vi "Host_Laser.vi"() -> ()   [LabVIEW 2018]
uses:
  <vilib>/userdefined/High Color/nirio_resource_hc.ctl
  C:/LabView_PRJ/EV76C661/Spels.AutomationTools.RemoteFunctionalControlService.dll
  Spels.AutomationTools.RemoteFunctionalControlService.dll
  <instrlib>/niDCPower/nidcpower.llb/niDCPower Measurement Type.ctl
  <vilib>/FPGAPlugInAG/PXI-7953R/niLvFpga_Open_PXI-7953R.vi
  <vilib>/rvi/interface/common/dynamic/niFpgaDynamicAddResources.vi
  <vilib>/FPGAPlugInAG/Dynamic/niLvFpga_Reset_Dynamic.vi
  <vilib>/FPGAPlugInAG/Dynamic/niLvFpga_Run_Dynamic.vi
  <vilib>/Utility/error.llb/Error Cluster From Error Code.vi
  <vilib>/rvi/errors/niLvFpgaAdjustHostInterfaceError.vi
  <vilib>/FPGAPlugInAG/Dynamic/niLvFpga_Abort_Dynamic.vi
  <vilib>/rvi/interface/nirviOpenFPGA/nirviOpenFPGA.xnode
  FPGA Bitfiles/EV76C661_FPGATarget_Target_LxE3WAGXilk.lvbitx
  <vilib>/rvi/interface/nirviMethod/nirviMethod.xnode
  <vilib>/rvi/interface/nirviReadWriteControl/nirviReadWriteControl.xnode
  NiFpgaLv.dll
  <vilib>/rvi/interface/Simulation/niFpgaSimulationCallBeginRW.vi
  <vilib>/FPGAPlugInAG/Dynamic/niLvFpga_ReadFifo_Dynamic.vi
  <vilib>/rvi/errors/niLvFpgaMergeErrorWithErrorCode.vi
panel:
  out "Data":string
  out "Image":T1(plugin-control)
  in  "Содержание всех регистров":u32[](array[numeric])=[1, 0, 0, 0, 32880, 0, 53338, 2561, 56217, 24976, 512, 260, 0, 0, 512, 0, 0, 0, 6, 1024, 6, 1280, 0, 0, 0, 0, 0, 512, 0, 0, 0, 6, 1024, 6, 1280, 0, 512, 0, 0, 0, 6, 1024, 6, 1280, 0, 512, 0, 0, 0, 6, 1024, 6, 1280, 0, 32896, 32896, 0, 14464, 32960, 0, 0, 0, 0, 0, 0, 0, 0, 0, 8192, 0, 0, 0, 0, 31601, 0, 0, 0, 0, 0, 0, 0, 0, 0, 0, 0, 0, 0, 0, 0, 0, 0, 0, 0, 0, 0, 0, 0, 0, 0, 0, 0, 0, 0, 0, 0, 0, 0, 0, 0, 0, 0, 0, 0, 0, 0, 0, 0, 0, 0, 0, 0, 0, 0, 0, 0, 0, 0, 2048]
  in  "Запись 6 регистров":u32[](array[numeric])=[2561, 56217, 24976, 512, 260, 512]
  in  "SPI_прошить":bool
  out "ST":bool
  in  "RESET":bool
  in  "Автомат":bool
  in  "VDD33_ON":bool
  in  "VDD18_ON":bool
  in  "Светлый (T)\nТемный (F)":bool
  in  "Frames":path=path "C:/LabView_PRJ/EV76C661/FRAMES"
  in  "ПРИМЕЧАНИЕ":string
  in  "SAVE":bool
  in  "Получить кадр":bool
  out "Data":u8[][](array[numeric])
  in  "Непрерывно":bool
  out "Сбои":i32
  out "СБОЙ":string="ОК"
  out "СБОЙ!":bool
  out "ПОСЛЕДНИЙ СБОЙ":string="0"
  out "COUNT":u8
  out "SPI_OUT":bool[](array[boolean])
  in  "МАСКИРУЕМ":i32[](array[numeric])=[0, -1, 2, 3, 4, 5, 6, 7, 8, 9, 10, 11, 12, 13, 14, 15, 16, 17, 18, 19, 20, 21, 22, 23, 24, 25, 26, 27, 28, 29, 30, 31, 32, 33, 34, 35, 36, 37, 38, 39, 40, 41, 42, 43, 44, 45, 46, 47, 48, 49, 50, 51, 52, 53, 54, 55, 56, 57, 58, 59, -1, -1, -1, -1, -1, -1, -1, -1, -1, -1, -1, -1, -1, -1, -1, -1, -1, -1, -1, -1, -1, -1, -1, -1, -1, -1, -1, -1, -1, -1, -1, -1, -1, -1, -1, -1, -1, -1, -1, -1, -1, -1, -1, -1, -1, -1, -1, -1, -1, -1, -1, -1, -1, -1, -1, -1, -1, -1, -1, -1, -1, -1, -1, -1, -1, -1, -1, 127, 0, 0, 0, 0, 0, 0, 0, 0, 0, 0, 0, 0, 0, 0, 0, 0, 0, 0, 0, 0, 0, 0, 0, 0, 0, 0, 0, 0, 0, 0, 0, 0, 0, 0, 0, 0, 0, 0, 0, 0, 0, 0, 0, 0, 0, 0, 0, 0, 0, 0, 0, 0, 0, 0, 0, 0, 0, 0, 0, 0, 0, 0, 0, 0, 0, 0, 0, 0, 0, 0, 0, 0, 0, 0, 0, 0, 0, 0, 0, 0, 0, 0, 0, 0, 0, 0, 0, 0, 0, 0, 0, 0, 0, 0, 0, 0, 0, 0, 0, 0, 0, 0, 0, 0, 0, 0, 0, 0, 0, 0, 0, 0, 0, 0, 0, 0, 0, 0, 0, 0, 0, 0, 0, 0, 0, 0, 0, 0]
  in  "ПРОВЕРКА СБОЕВ?":bool
  out "GC":u8
  out "REG_WR":bool
  in  "SIM_SEL":bool
  out "SEL":bool
  in  "VDD18A_selcur":dbl=0.05 caption="current limit" format="%_6p"
  in  "VDD33A_selcur":dbl=0.035 caption="current limit" format="%_6p"
  in  "VDD18D_selcur":dbl=0.055 caption="current limit" format="%_6p"
  out "VDD18A":i32
  out "VDD18A":bool
  out "VDD33A":i32
  out "VDD33A":bool
  out "VDD18D":i32
  out "VDD18D":bool
  in  "VDD18A, V":dbl=1.8 caption="voltage level" format="%_6p"
  in  "VDD18A_curlim, A":dbl=0.1 caption="current limit" format="%_6p"
  in  "VDD33A_curlim, A":dbl=0.1 caption="current limit" format="%_6p"
  out "VDD18A_cur, A":dbl caption="measurement" format="%_6g"
  out "VDD33A_cur, A":dbl caption="measurement" format="%_6g"
  in  "VDD33A, V":dbl=3.3 caption="voltage level" format="%_6p"
  in  "VDD18D, V":dbl=1.8 caption="voltage level" format="%_6p"
  in  "VDD18D_curlim, A":dbl=0.1 caption="current limit" format="%_6p"
  out "VDD18D_cur, A":dbl caption="measurement" format="%_6g"
  in  "Питание":bool
  out "VDD33A Chart":dbl(graph)=0.0006520018718277456
  out "VDD18D Chart":dbl(graph)=-6.889343232631937
  out "VDD18A Chart":dbl(graph)=0.09491557293549348 caption="Waveform Chart 5"
  in  "Стоп":bool
  in  "VDD18A_33A":refnum<k15>="PXI1Slot2" caption="instrument handle"
  in  "VDD18D":refnum<k15>="PXI1Slot3" caption="instrument handle"
  in  "resource name":T2="PXI1Slot6"
  in  "SEU":path=path "C:/LabView_PRJ/EV76C661/SEU"
  in  "SEL":path=path "C:/LabView_PRJ/EV76C661/SEL"
  out "Номер образца":string="0"
  # "1,6/1,8/2,0"
  # "3,15/3,3/3,45"
  # "h07, h08, h09, h0A, h0B, h0E"
  # "h0E - отвечает за экспозицию\nОт 1 до 65535"
  # "1,6/1,8/2,0"
  # "0"
  # "1"
  # "2"
  # "3"
  # "4"
  # "5"
  # "6"
  # "7"
  # "8"
  # "9"
  # "10"
  # "11"
  # "12"
  # "13"
  # "14"
  # "15"
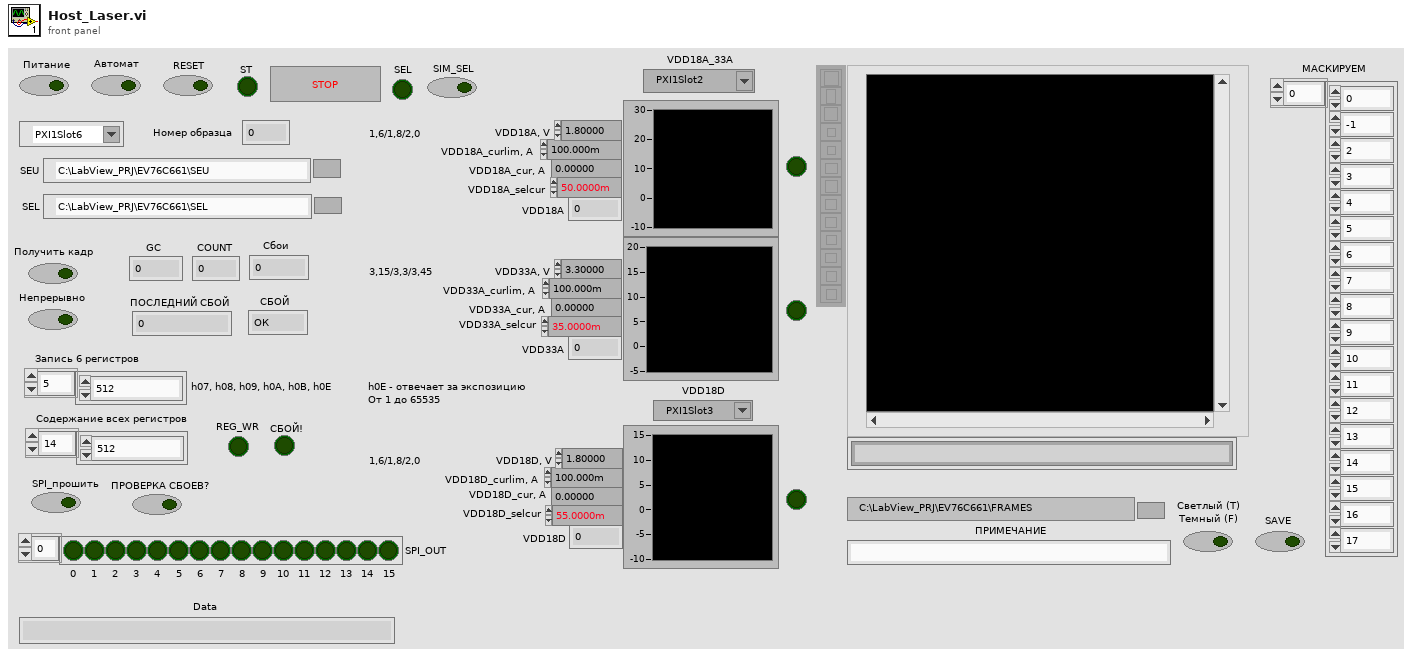
[diagram p1: front panel]
types:
  T1 = typedef "IMAQ Image.ctl" = refnum<image>
  T2 = typedef "nirio_resource_hc.ctl" = tag
  T3 = typedef "Image Type" = u32
  T4 = enum16{"open", "replace", "create", "open or create", "replace or create", "replace or create with confirmation"}
  T5 = typedef "niDCPower Measurement Type.ctl" = i32
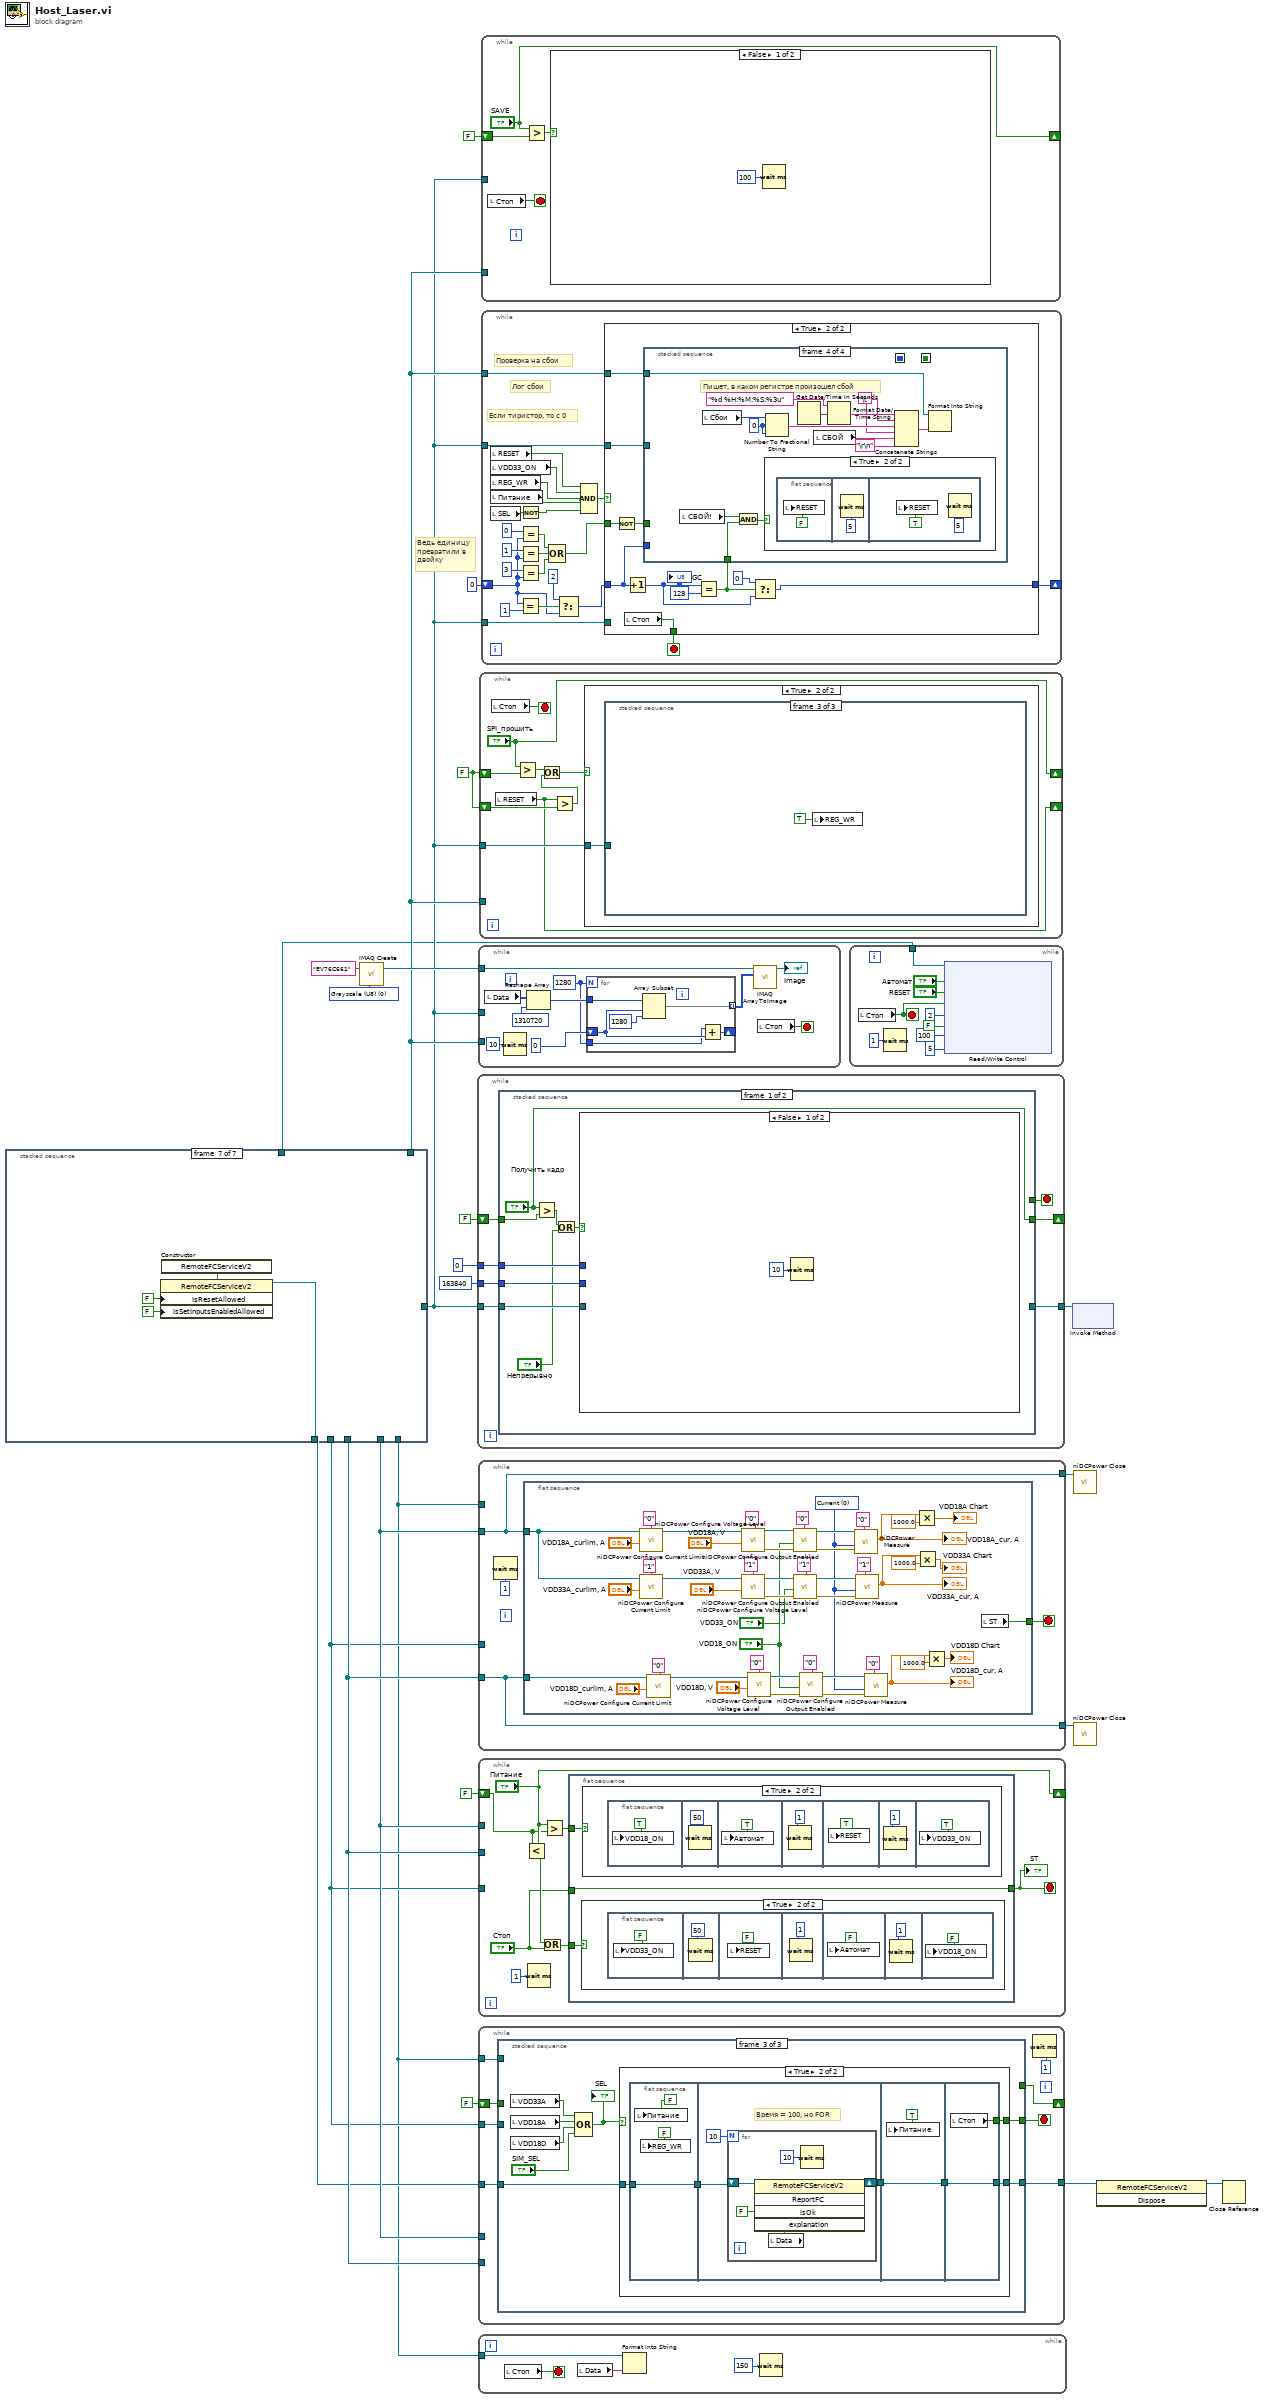
[diagram p0: block diagram]
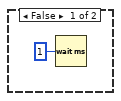
[diagram p2: hidden frame]
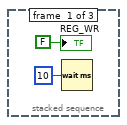
[diagram p3: hidden frame]
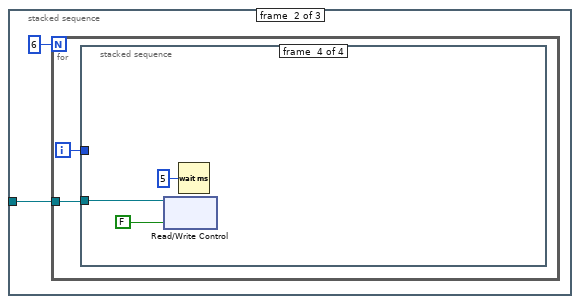
[diagram p4: hidden frame]
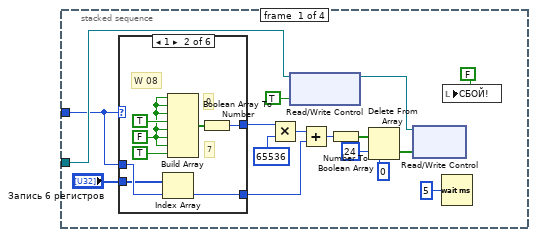
[diagram p5: hidden frame]
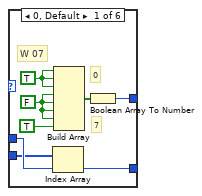
[diagram p6: hidden frame]
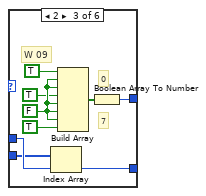
[diagram p7: hidden frame]
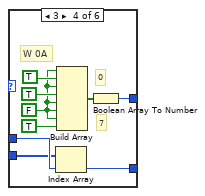
[diagram p8: hidden frame]
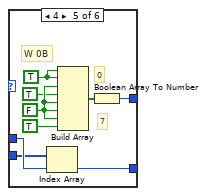
[diagram p9: hidden frame]
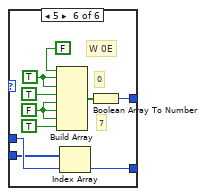
[diagram p10: hidden frame]
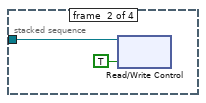
[diagram p11: hidden frame]
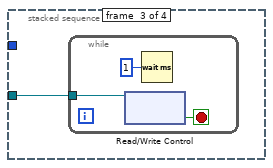
[diagram p12: hidden frame]
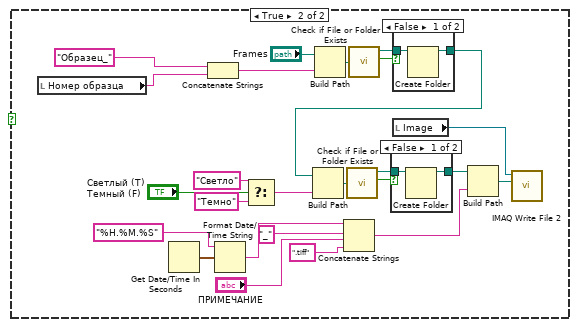
[diagram p15: hidden frame]
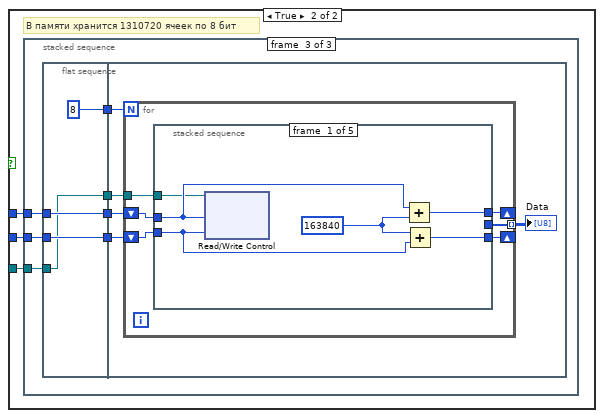
[diagram p18: hidden frame]
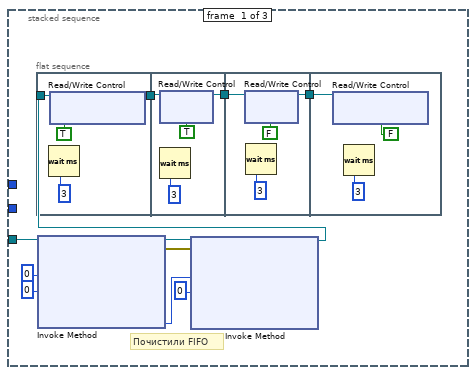
[diagram p19: hidden frame]
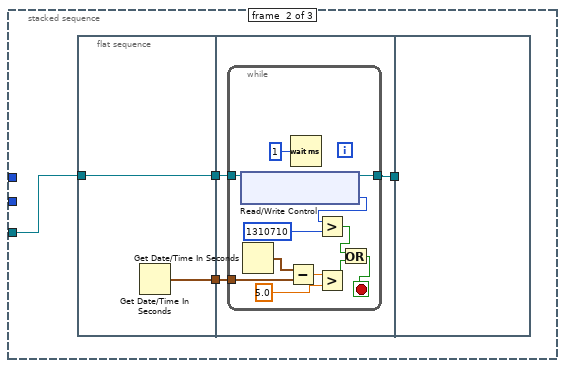
[diagram p20: hidden frame]
diagram:
  w7 = FALSE
  w19 = T3 0 items=["Grayscale (U8)", "Grayscale (I16)", "Grayscale (SGL)", "Complex (CSG)", "RGB (U32)", "HSL (U32)", "RGB (U64)"] ("Image Type")
  # "Ведь единицу \nпревратили в \nдвойку"
  n1 = stacked-sequence {
    tunnel: [_ _ _ _ w95 _ _] -> w6
    tunnel: [_ _ _ _ _ w102 _] -> w12
    tunnel: [_ _ _ _ _ w101 _] -> w11
    tunnel: [_ _ w40 _ _ _ _] -> w3
    tunnel: [_ _ _ _ w95 _ _] -> w10
    tunnel: [_ _ _ w66 _ _ _] -> w9
    tunnel: [_ _ _ _ w95 _ _] -> w5
    tunnel: [_ _ _ _ _ _ w113] -> w4
    frame #0 {
      n2 = call "Begin.vi"() -> ("Номер образца 2"=→"Номер образца":string)  [unwired: 11 in]
    }
    frame #1 {
      w29 = 0
      w30 = ""
      w26 = FALSE
      n3 = local write "ПОСЛЕДНИЙ СБОЙ"(w30) -> ()
      n4 = local write "СБОЙ"(w30) -> ()
      n5 = local write "Сбои"(w29) -> ()
      n6 = local write "VDD18A"(w29) -> ()
      n7 = local write "VDD33A"(w29) -> ()
      n8 = local write "VDD18D"(w29) -> ()
      n9 = local write "GC"(u8 0 ("GC")) -> ()
      n10 = local write "COUNT"(u16 0 ("COUNT")) -> ()
      n11 = local write "RESET"(w26) -> ()
      n12 = local write "SPI_прошить"(w26) -> ()
      n13 = local write "REG_WR"(w26) -> ()
      n14 = local write "Непрерывно"(w26) -> ()
      n15 = local write "Получить кадр"(w26) -> ()
      n16 = local write "VDD18A"(w26) -> ()
      n17 = local write "VDD33A"(w26) -> ()
      n18 = local write "VDD18D"(w26) -> ()
      n19 = local write "ST"(w26) -> ()
      n20 = local write "SEL"(w26) -> ()
      n21 = local write "Питание"(w26) -> ()
      n22 = local write "Стоп"(w26) -> ()
      n23 = local write "СБОЙ!"(w26) -> ()
      n24 = local write "SAVE"(w26) -> ()
      n25 = local write "ПРОВЕРКА СБОЕВ?"(w26) -> ()
      n26 = local write "Автомат"(w26) -> ()
      n27 = local write "SIM_SEL"(w26) -> ()
      n28 = local write "VDD18_ON"(w26) -> ()
      n29 = local write "VDD33_ON"(w26) -> ()
    }
    frame #2 {
      w41 = "\t"
      # "Инициализаци первой строки лога по токам"
      n30 = local read "Номер образца"() -> (w53:string)
      n31 = Build Path(base path="SEL", name or relative path=w53) -> (appended path=w55:path)
      n32 = Get Date/Time In Seconds() -> (seconds since 1Jan1904=w48:timestamp)
      n33 = call <vilib>:"Check if File or Folder Exists.vi"("path"=w55) -> ("file or folder exists?"=w56:bool, "dup path"=w57:path)  [unwired: 8 in, 1 out]
      n34 = Format Date/Time String(time format string (%c)="%d %H.%M.%S", seconds (now)=w48) -> (date/time string=w45:string)  [unwired: 1 in]
      n35 = case shown="False" w56 {
        tunnel: w57 -> [w63 w64]
        tunnel: [w62 w64] -> w39
        frame False {
          n36 = Create Folder(path (use dialog)=w63) -> (created path=w62:path)  [unwired: 2 in, 2 out]
        }
        frame True {
        }
      }
      n37 = Concatenate Strings(w45, ".xls" ("string")) -> (w43:string)
      n38 = Build Path(base path=w39, name or relative path=w43) -> (appended path=w46:path)
      n39 = Open/Create/Replace File(file path (use dialog)=w46, operation (0:open)=T4."open or create", access (0:read/write)=enum16{"read/write", "read-only", "write-only"}."read/write") -> (refnum out=w49:refnum<file>)  [unwired: 3 in, 2 out]
      n40 = case shown="True" TRUE {
        tunnel: w49 -> [w58 w61]
        tunnel: [w58 w59] -> w42
        frame False {
        }
        frame True {
          n41 = Set File Position(refnum=w61, from (0:start)=enum16{"start", "end", "current"}."end") -> (refnum out=w59:refnum<file>)  [unwired: 2 in, 1 out]
        }
      }
      n42 = Format Into String(initial string=w42, "Time" ("input 1"), w41, "V_18A_cur" ("input 1"), w41, "V_33A_cur" ("input 1"), w41, "V_18D_cur" ("input 1"), w41, "V_18A_sel" ("input 1"), w41, "V_33A_sel" ("input 1"), w41, "V_18D_sel" ("input 1"), "\r\n") -> (resulting string=w40:refnum<file>)  [unwired: 2 in, 1 out]
    }
    frame #3 {
      w75 = "\t"
      n43 = local read "Номер образца"() -> (w83:string)
      n44 = Build Path(base path="SEU", name or relative path=w83) -> (appended path=w85:path)
      n45 = Get Date/Time In Seconds() -> (seconds since 1Jan1904=w81:timestamp)
      n46 = call <vilib>:"Check if File or Folder Exists.vi"("path"=w85) -> ("file or folder exists?"=w86:bool, "dup path"=w87:path)  [unwired: 8 in, 1 out]
      n47 = Format Date/Time String(time format string (%c)="%d %H.%M.%S", seconds (now)=w81) -> (date/time string=w79:string)  [unwired: 1 in]
      n48 = case shown="False" w86 {
        tunnel: w87 -> [w93 w94]
        tunnel: [w92 w94] -> w65
        frame False {
          n49 = Create Folder(path (use dialog)=w93) -> (created path=w92:path)  [unwired: 2 in, 2 out]
        }
        frame True {
        }
      }
      n50 = Concatenate Strings(w79, ".xls" ("string")) -> (w78:string)
      n51 = Build Path(base path=w65, name or relative path=w78) -> (appended path=w80:path)
      n52 = Open/Create/Replace File(file path (use dialog)=w80, operation (0:open)=T4."open or create", access (0:read/write)=enum16{"read/write", "read-only", "write-only"}."read/write") -> (refnum out=w82:refnum<file>)  [unwired: 3 in, 2 out]
      n53 = case shown="True" TRUE {
        tunnel: w82 -> [w88 w91]
        tunnel: [w88 w89] -> w77
        frame False {
        }
        frame True {
          n54 = Set File Position(refnum=w91, from (0:start)=enum16{"start", "end", "current"}."end") -> (refnum out=w89:refnum<file>)  [unwired: 2 in, 1 out]
        }
      }
      n55 = Format Into String(initial string=w77, "Time" ("input 1"), w75, "Count" ("input 3"), w75, "#reg" ("input 5"), "\r\n") -> (resulting string=w66:refnum<file>)  [unwired: 2 in, 1 out]
    }
    frame #4 {
      n56 = xnode "Open FPGA VI Reference"("resource name"="resource name") -> ("FPGA VI Reference Out"=w100:refnum<k20>, "error out"=w98:errorcluster)  [unwired: 1 in]
      n57 = xnode "Invoke Method"("FPGA VI Reference In"=w100, "error in"=w98) -> ("FPGA VI Reference Out"=w97:refnum<k20>, "error out"=w99:errorcluster)
      n58 = xnode "Invoke Method"("FPGA VI Reference In"=w97, "error in"=w99) -> ("FPGA VI Reference Out"=w95:refnum<k20>)  [unwired: 1 in, 1 out]
    }
    frame #5 {
      n59 = call <instrlib>:"niDCPower Initialize.vi"("resource name"="VDD18A_33A") -> ("error out"=w109:errorcluster, "instrument handle out"=w111:refnum<k15>)  [unwired: 3 in, 6 out]
      n60 = call <instrlib>:"niDCPower Initialize.vi"("resource name"="VDD18D") -> ("error out"=w110:errorcluster, "instrument handle out"=w112:refnum<k15>)  [unwired: 3 in, 6 out]
      n61 = call <instrlib>:"niDCPower Configure Voltage Level.vi"("error in (no error)"=w109, "voltage level"=0.0, "channel name"="0,1", "instrument handle"=w111) -> ("instrument handle out"=w101:refnum<k15>)  [unwired: 6 in, 1 out]
      n62 = call <instrlib>:"niDCPower Configure Voltage Level.vi"("error in (no error)"=w110, "voltage level"=0.0, "channel name"="0", "instrument handle"=w112) -> ("instrument handle out"=w102:refnum<k15>)  [unwired: 6 in, 1 out]
    }
    frame #6 {
      n63 = constructor class="RemoteFCServiceV2"() -> (reference out=w116:refnum<k24>)  [unwired: 3 in, 2 out]
      n64 = property class="RemoteFCServiceV2"(reference=w116, "IsResetAllowed"=FALSE, "IsSetInputsEnabledAllowed"=FALSE) -> (reference out=w113:refnum<k24>)  [unwired: 1 in, 1 out]
    }
  }
  n65 = call "IMAQ Create"("Image Name"="EV76C661", "Image Type"=w19) -> ("New Image"=w18:T1)  [unwired: 3 in, 1 out]
  n66 = while {
    tunnel: w6 -> [w123]
    tunnel: [w122] -> w24
    tunnel: u32 163840 ("163840") -> [w121]
    tunnel: u32 0 -> [w119]
    shift-right: [w117] -> _
    shift-left: FALSE ("Получить кадр") -> [w118]
    stop <- w120 stop-if-true
    n67 = stacked-sequence {
      tunnel: w123 -> [w130 w227]
      tunnel: [_ w227] -> w122
      tunnel: w121 -> [w131 _]
      tunnel: [_ w226] -> w120
      tunnel: w119 -> [w129 _]
      tunnel: w118 -> [w128 _]
      tunnel: ["Получить кадр" _] -> w117
      frame #0 {
        n68 = Greater?(x="Получить кадр", y=w128) -> (0:w127:bool)
        n69 = Or(x=w127, y="Непрерывно") -> (x .or. y?=w125:bool)
        n70 = case shown="False" w125 {
          tunnel: w130 -> [_ w135]
          tunnel: w131 -> [_ w134]
          tunnel: w129 -> [_ w133]
          frame False {
            n71 = Wait (ms)(milliseconds to wait=u32 10) -> ()  [unwired: 1 out]
          }
          frame True {
            # "В памяти хранится 1310720 ячеек по 8 бит"
            n72 = stacked-sequence {
              tunnel: w135 -> [w140 w163 w189]
              tunnel: w134 -> [_ _ w185]
              tunnel: w133 -> [_ _ w187]
              frame #0 {
                # "Почистили FIFO"
                n73 = flat-sequence {
                  tunnel: w138 -> [w150]
                  tunnel: [w147] -> w139
                  tunnel: w139 -> [w152]
                  tunnel: [w151] -> w137
                  tunnel: w137 -> [w158]
                  tunnel: [w157] -> w136
                  tunnel: w136 -> [w161]
                  frame #0 {
                    n74 = Wait (ms)(milliseconds to wait=u32 3) -> ()  [unwired: 1 out]
                    n75 = xnode "Read/Write Control"("FPGA VI Reference In"=w150, "Кадр в память"=TRUE) -> ("FPGA VI Reference Out"=w147:refnum<k20>)  [unwired: 1 in, 1 out]
                  }
                  frame #1 {
                    n76 = xnode "Read/Write Control"("FPGA VI Reference In"=w152, "TRIG"=TRUE ("Кадр в память")) -> ("FPGA VI Reference Out"=w151:refnum<k20>)  [unwired: 1 in, 1 out]
                    n77 = Wait (ms)(milliseconds to wait=u32 3) -> ()  [unwired: 1 out]
                  }
                  frame #2 {
                    n78 = xnode "Read/Write Control"("FPGA VI Reference In"=w158, "TRIG"=FALSE) -> ("FPGA VI Reference Out"=w157:refnum<k20>)  [unwired: 1 in, 1 out]
                    n79 = Wait (ms)(milliseconds to wait=u32 3) -> ()  [unwired: 1 out]
                  }
                  frame #3 {
                    n80 = xnode "Read/Write Control"("FPGA VI Reference In"=w161, "Кадр в память"=FALSE ("Кадр на ПК")) -> ()  [unwired: 1 in, 2 out]
                    n81 = Wait (ms)(milliseconds to wait=u32 3) -> ()  [unwired: 1 out]
                  }
                }
                n82 = xnode "Invoke Method"("FPGA VI Reference In"=w140, "Number of Elements"=u32 0, "Timeout (ms)"=0) -> ("FPGA VI Reference Out"=w146:refnum<k20>, "error out"=w145:errorcluster, "Elements Remaining"=w144:u32)  [unwired: 1 in, 1 out]
                n83 = xnode "Invoke Method"("FPGA VI Reference In"=w146, "error in"=w145, "Number of Elements"=w144, "Timeout (ms)"=0) -> ("FPGA VI Reference Out"=w138:refnum<k20>)  [unwired: 3 out]
              }
              frame #1 {
                n84 = flat-sequence {
                  tunnel: w163 -> [w166]
                  tunnel: [w166] -> w165
                  tunnel: [w167] -> w162
                  tunnel: w165 -> [w170]
                  tunnel: [w169] -> w164
                  tunnel: w162 -> [w168]
                  tunnel: w164 -> [_]
                  frame #0 {
                    n85 = Get Date/Time In Seconds() -> (seconds since 1Jan1904=w167:timestamp)
                  }
                  frame #1 {
                    n86 = while {
                      tunnel: [w181] -> w169
                      tunnel: w170 -> [w180]
                      tunnel: w168 -> [w177]
                      stop <- w172 stop-if-true
                      n87 = xnode "Read/Write Control"("FPGA VI Reference In"=w180) -> ("FPGA VI Reference Out"=w181:refnum<k20>, "Записали адресов"=w171:u32)  [unwired: 1 in, 1 out]
                      n88 = Get Date/Time In Seconds() -> (seconds since 1Jan1904=w178:timestamp)
                      n89 = Subtract(x=w178, y=w177) -> (x-y=w176:dbl)
                      n90 = Wait (ms)(milliseconds to wait=u32 1) -> ()  [unwired: 1 out]
                      n91 = Greater?(x=w171, y=u32 1310710) -> (0:w174:bool)
                      n92 = Greater?(x=w176, y=5.0) -> (0:w173:bool)
                      n93 = Or(x=w174, y=w173) -> (x .or. y?=w172:bool)
                    }
                  }
                  frame #2 {
                  }
                }
              }
              frame #2 {
                n94 = flat-sequence {
                  tunnel: w189 -> [w190]
                  tunnel: [w193] -> w188
                  tunnel: w187 -> [w193]
                  tunnel: [w192] -> w186
                  tunnel: w185 -> [w192]
                  tunnel: [8 ("For FIFO")] -> w184
                  tunnel: [w190] -> w183
                  tunnel: w188 -> [w198]
                  tunnel: w186 -> [w197]
                  tunnel: w184 -> [w196]
                  tunnel: w183 -> [w195]
                  frame #0 {
                  }
                  frame #1 {
                    n95 = for {
                      N: w196 -> [_]
                      shift-right: [w202] -> _
                      shift-left: w198 -> [w204]
                      shift-right: [w201] -> _
                      shift-left: w197 -> [w203]
                      tunnel: w195 -> [w200]
                      tunnel: [w199] -> w194 mode=indexing
                      n96 = stacked-sequence {
                        tunnel: [_ _ _ _ w223] -> w199
                        tunnel: [w210 _ _ _ _] -> w202
                        tunnel: [w209 _ _ _ _] -> w201
                        tunnel: w204 -> [w207 _ _ _ _]
                        tunnel: w203 -> [w208 _ _ _ _]
                        tunnel: w200 -> [w206 w211 w213 w215 w222]
                        frame #0 {
                          w205 = u32 163840 ("163840")
                          n97 = xnode "Read/Write Control"("FPGA VI Reference In"=w206, "Нач_адр"=w207, "Кон_адр"=w208) -> ()  [unwired: 1 in, 2 out]
                          n98 = Add(x=w207, y=w205) -> (x+y=w210:u32)
                          n99 = Add(x=w205, y=w208) -> (x+y=w209:u32)
                        }
                        frame #1 {
                          n100 = xnode "Read/Write Control"("FPGA VI Reference In"=w211, "Кадр на ПК"=TRUE ("HOST")) -> ()  [unwired: 1 in, 2 out]
                        }
                        frame #2 {
                          n101 = xnode "Read/Write Control"("FPGA VI Reference In"=w213, "Кадр на ПК"=FALSE ("HOST")) -> ()  [unwired: 1 in, 2 out]
                        }
                        frame #3 {
                          n102 = while {
                            tunnel: w215 -> [w216]
                            stop <- w218 stop-if-true
                            # "Записан FIFO?"
                            n103 = xnode "Read/Write Control"("FPGA VI Reference In"=w216) -> ("Записали FIFO"=w218:bool)  [unwired: 1 in, 2 out]
                            n104 = Wait (ms)(milliseconds to wait=u32 1) -> ()  [unwired: 1 out]
                          }
                        }
                        frame #4 {
                          n105 = xnode "Invoke Method"("FPGA VI Reference In"=w222, "Number of Elements"=u32 0, "Timeout (ms)"=0) -> ("FPGA VI Reference Out"=w224:refnum<k20>, "Elements Remaining"=w225:u32)  [unwired: 1 in, 2 out]
                          n106 = xnode "Invoke Method"("FPGA VI Reference In"=w224, "Number of Elements"=w225, "Timeout (ms)"=0) -> ("Data"=w223:u8[])  [unwired: 1 in, 3 out]
                        }
                      }
                    }
                    "Data" <- w194
                  }
                }
              }
            }
          }
        }
      }
      frame #1 {
        n107 = local read "Стоп"() -> (w226:bool)
      }
    }
  }
  n108 = while {
    tunnel: w18 -> [w234]
    tunnel: w6 -> [_]
    tunnel: w9 -> [_]
    stop <- w237 stop-if-true
    w228 = 1280 ("length")
    n109 = local read "Data"() -> (w235:u8[][])
    n110 = Wait (ms)(milliseconds to wait=u32 10) -> ()  [unwired: 1 out]
    n111 = Reshape Array(w235, 1310720 ("dimension size")) -> (w232:u8[])
    n112 = for {
      N: w228 -> [_]
      tunnel: w232 -> [w243]
      shift-right: [w242] -> _
      shift-left: 0 ("index") -> [w241]
      tunnel: [w240] -> w230 mode=indexing
      tunnel: w228 -> [w239]
      n113 = Array Subset(array=w243, index=w241, length=1280) -> (w240:u8[])
      n114 = Add(x=w239, y=w241) -> (x+y=w242:i32)
    }
    n115 = call "IMAQ ArrayToImage"("Image Pixels (U8)"=w230, "Image"=w234) -> ("Image Out"=→"Image":T1)  [unwired: 8 in, 1 out]
    n116 = local read "Стоп"() -> (w237:bool)
  }
  n117 = while {
    shift-right: ["Питание"] -> _
    shift-left: FALSE -> [w250]
    tunnel: w10 -> [_]
    tunnel: w12 -> [_]
    tunnel: w11 -> [_]
    stop <- w244 stop-if-true
    n118 = Less?(x="Питание", y=w250) -> (x < y?=w246:bool)
    n119 = Wait (ms)(milliseconds to wait=u32 1) -> ()  [unwired: 1 out]
    n120 = Or(x=w246, y="Стоп") -> (x .or. y?=w247:bool)
    n121 = Greater?(x="Питание", y=w250) -> (0:w249:bool)
    n122 = flat-sequence {
      tunnel: w247 -> [w254]
      tunnel: w249 -> [w253]
      tunnel: [w252] -> w244
      tunnel: "Стоп" -> [w252]
      frame #0 {
        n123 = case shown="True" w254 {
          frame False {
          }
          frame True {
            n124 = flat-sequence {
              frame #0 {
                n125 = local write "VDD33_ON"(FALSE ("VDD18_ON")) -> ()
              }
              frame #1 {
                n126 = Wait (ms)(milliseconds to wait=u32 50) -> ()  [unwired: 1 out]
              }
              frame #2 {
                n127 = local write "RESET"(FALSE ("Автомат")) -> ()
              }
              frame #3 {
                n128 = Wait (ms)(milliseconds to wait=u32 1) -> ()  [unwired: 1 out]
              }
              frame #4 {
                n129 = local write "Автомат"(FALSE ("RESET")) -> ()
              }
              frame #5 {
                n130 = Wait (ms)(milliseconds to wait=u32 1) -> ()  [unwired: 1 out]
              }
              frame #6 {
                n131 = local write "VDD18_ON"(FALSE ("VDD33_ON")) -> ()
              }
            }
          }
        }
        n132 = case shown="True" w253 {
          frame False {
          }
          frame True {
            n133 = flat-sequence {
              frame #0 {
                n134 = local write "VDD18_ON"(TRUE ("VDD18_ON")) -> ()
              }
              frame #1 {
                n135 = Wait (ms)(milliseconds to wait=u32 50) -> ()  [unwired: 1 out]
              }
              frame #2 {
                n136 = local write "Автомат"(TRUE ("Автомат")) -> ()
              }
              frame #3 {
                n137 = Wait (ms)(milliseconds to wait=u32 1) -> ()  [unwired: 1 out]
              }
              frame #4 {
                n138 = local write "RESET"(TRUE ("RESET")) -> ()
              }
              frame #5 {
                n139 = Wait (ms)(milliseconds to wait=u32 1) -> ()  [unwired: 1 out]
              }
              frame #6 {
                n140 = local write "VDD33_ON"(TRUE ("VDD33_ON")) -> ()
              }
            }
          }
        }
      }
    }
    "ST" <- w244
  }
  n141 = while {
    shift-right: [w275] -> _
    shift-left: FALSE -> [w274]
    tunnel: w10 -> [w273]
    tunnel: w3 -> [w272]
    tunnel: w12 -> [_]
    tunnel: w11 -> [_]
    tunnel: w4 -> [w270]
    tunnel: [w269] -> w2
    stop <- w271 stop-if-true
    n142 = stacked-sequence {
      tunnel: [w277 _ _] -> w275
      tunnel: w274 -> [w278 _ _]
      tunnel: w273 -> [_ _ _]
      tunnel: w272 -> [_ _ _]
      tunnel: [_ _ w327] -> w271
      tunnel: w270 -> [_ _ w326]
      tunnel: [_ _ w325] -> w269
      frame #0 {
        # "Проверка токов на тиристоры"
        n143 = flat-sequence {
          tunnel: w279 -> [w280]
          frame #0 {
            n144 = case shown="True" w280 {
              frame False {
              }
              frame True {
                n145 = Wait (ms)(milliseconds to wait=u32 500) -> ()  [unwired: 1 out]
              }
            }
          }
          frame #1 {
            n146 = local read "VDD18A_cur, A"() -> (w284:dbl)
            n147 = local read "VDD18D_cur, A"() -> (w282:dbl)
            n148 = local read "VDD33A_cur, A"() -> (w283:dbl)
            n149 = Greater?(x=w282, y="VDD18D_selcur") -> (0:w285:bool)
            "VDD18D" <- w285
            n150 = Greater?(x=w284, y="VDD18A_selcur") -> (0:w289:bool)
            "VDD18A" <- w289
            n151 = Greater?(x=w283, y="VDD33A_selcur") -> (0:w287:bool)
            "VDD33A" <- w287
            n152 = case shown="True" w289 {
              frame False {
              }
              frame True {
                n153 = local read "VDD18A"() -> (w296:i32)
                n154 = Increment(x=w296) -> (x+1=→"VDD18A":i32)
              }
            }
            n155 = case shown="True" w287 {
              frame False {
              }
              frame True {
                n156 = local read "VDD33A"() -> (w293:i32)
                n157 = Increment(x=w293) -> (x+1=→"VDD33A":i32)
              }
            }
            n158 = case shown="True" w285 {
              frame False {
              }
              frame True {
                n159 = local read "VDD18D"() -> (w292:i32)
                n160 = Increment(x=w292) -> (x+1=→"VDD18D":i32)
              }
            }
          }
        }
        n161 = local read "Питание"() -> (w277:bool)
        n162 = Greater?(x=w277, y=w278) -> (0:w279:bool)
      }
      frame #1 {
        w314 = i16 0 ("width (-)")
        w315 = i16 3 ("width (-)")
        w306 = "\t"
        n163 = local read "VDD18A_cur, A"() -> (w303:dbl)
        n164 = local read "VDD33A_cur, A"() -> (w302:dbl)
        n165 = local read "VDD18D_cur, A"() -> (w301:dbl)
        n166 = local read "VDD18A"() -> (w300:i32)
        n167 = local read "VDD33A"() -> (w299:i32)
        n168 = local read "VDD18D"() -> (w298:i32)
        n169 = Number To Fractional String(number=w303, width (-)=w315, precision (6)=w315) -> (F-format string=w313:string)  [unwired: 1 in]
        n170 = Number To Fractional String(number=w302, width (-)=w315, precision (6)=w315) -> (F-format string=w312:string)  [unwired: 1 in]
        n171 = Number To Fractional String(number=w301, width (-)=w315, precision (6)=w315) -> (F-format string=w311:string)  [unwired: 1 in]
        n172 = Number To Fractional String(number=w300, width (-)=w314, precision (6)=w314) -> (F-format string=w309:string)  [unwired: 1 in]
        n173 = Number To Fractional String(number=w299, width (-)=w314, precision (6)=w314) -> (F-format string=w308:string)  [unwired: 1 in]
        n174 = Number To Fractional String(number=w298, width (-)=w314, precision (6)=w314) -> (F-format string=w307:string)  [unwired: 1 in]
        n175 = Get Date/Time In Seconds() -> (seconds since 1Jan1904=w324:timestamp)
        n176 = Format Date/Time String(time format string (%c)="%d %H:%M:%S:%3u", seconds (now)=w324) -> (date/time string=w316:string)  [unwired: 1 in]
        n177 = local read "VDD33A"() -> (w320:bool)
        n178 = local read "VDD18A"() -> (w319:bool)
        n179 = local read "VDD18D"() -> (w318:bool)
        n180 = local read "SIM_SEL"() -> (w317:bool)
        n181 = Compound Arithmetic op=OR(w320, w319, w318, w317) -> (w310:bool)
        n182 = Select(t="!!!", s=w310, f="") -> (s? t:f=w305:string)
        n183 = Concatenate Strings(w316, w306, w313, w306, w312, w306, w311, w306, w309, w306, w308, w306, w307, w306, w306, w305, "\r\n") -> (→"Data":string)
      }
      frame #2 {
        n184 = local read "VDD33A"() -> (w332:bool)
        n185 = local read "VDD18A"() -> (w331:bool)
        n186 = local read "VDD18D"() -> (w330:bool)
        n187 = Compound Arithmetic op=OR(w332, w331, w330, "SIM_SEL") -> (w328:bool)
        "SEL" <- w328
        n188 = case shown="True" w328 {
          tunnel: [w336 w342] -> w327
          tunnel: w326 -> [w333 w340]
          tunnel: [w333 w337] -> w325
          frame False {
            n189 = local read "Data"() -> (w334:string)
            n190 = invoke class="RemoteFCServiceV2" method="ReportFC"(reference=w333, "isOk"=TRUE, "explanation"=w334) -> ()  [unwired: 2 in, 5 out]
            n191 = local read "Стоп"() -> (w336:bool)
          }
          frame True {
            n192 = flat-sequence {
              tunnel: [w343] -> w341
              tunnel: w340 -> [w343]
              tunnel: w341 -> [w348]
              tunnel: [w347] -> w338
              tunnel: [w354] -> w339
              tunnel: w338 -> [w354]
              tunnel: [w357] -> w342
              tunnel: w339 -> [w356]
              tunnel: [w356] -> w337
              frame #0 {
                n193 = local write "Питание"(FALSE ("SYS_RESET")) -> ()
                n194 = local write "REG_WR"(FALSE ("SYS_RESET")) -> ()
              }
              frame #1 {
                # "Время = 100, но FOR"
                n195 = for {
                  N: 10 -> [_]
                  shift-right: [w351] -> w347
                  shift-left: w348 -> [w353]
                  n196 = local read "Data"() -> (w352:string)
                  n197 = invoke class="RemoteFCServiceV2" method="ReportFC"(reference=w353, "isOk"=FALSE, "explanation"=w352) -> (reference out=w351:refnum<k24>)  [unwired: 2 in, 4 out]
                  n198 = Wait (ms)(milliseconds to wait=u32 10) -> ()  [unwired: 1 out]
                }
              }
              frame #2 {
                n199 = local write "Питание"(TRUE ("SYS_RESET")) -> ()
              }
              frame #3 {
                n200 = local read "Стоп"() -> (w357:bool)
              }
            }
          }
        }
      }
    }
    n201 = Wait (ms)(milliseconds to wait=u32 1) -> ()  [unwired: 1 out]
  }
  n202 = while {
    tunnel: w3 -> [w361]
    stop <- w358 stop-if-true
    n203 = local read "Стоп"() -> (w358:bool)
    n204 = local read "Data"() -> (w360:string)
    n205 = Format Into String(initial string=w361, w360) -> ()  [unwired: 2 in, 2 out]
    n206 = Wait (ms)(milliseconds to wait=u32 150) -> ()  [unwired: 1 out]
  }
  n207 = while {
    tunnel: w12 -> [w362]
    tunnel: w11 -> [w363]
    tunnel: [w363] -> w16
    tunnel: [w362] -> w15
    tunnel: w3 -> [_]
    tunnel: w10 -> [_]
    stop <- w364 stop-if-true
    n208 = Wait (ms)(milliseconds to wait=u32 1) -> ()  [unwired: 1 out]
    n209 = flat-sequence {
      tunnel: w363 -> [w371]
      tunnel: w362 -> [w370]
      tunnel: [w366] -> w364
      frame #0 {
        w381 = T5 0 items=["Current", "Voltage"] ("measurement type")
        n210 = call <instrlib>:"niDCPower Configure Current Limit.vi"("current limit"="VDD18A_curlim, A", "channel name"="0", "instrument handle"=w371) -> ("instrument handle out"=w403:refnum<k15>)  [unwired: 7 in, 1 out]
        n211 = call <instrlib>:"niDCPower Configure Current Limit.vi"("current limit"="VDD33A_curlim, A", "channel name"="1", "instrument handle"=w371) -> ("instrument handle out"=w404:refnum<k15>)  [unwired: 7 in, 1 out]
        n212 = call <instrlib>:"niDCPower Configure Current Limit.vi"("current limit"="VDD18D_curlim, A", "channel name"="0", "instrument handle"=w370) -> ("instrument handle out"=w386:refnum<k15>)  [unwired: 7 in, 1 out]
        n213 = call <instrlib>:"niDCPower Configure Voltage Level.vi"("voltage level"="VDD18A, V", "channel name"="0", "instrument handle"=w403) -> ("error out"=w396:errorcluster, "instrument handle out"=w399:refnum<k15>)  [unwired: 7 in]
        n214 = call <instrlib>:"niDCPower Configure Voltage Level.vi"("voltage level"="VDD33A, V", "channel name"="1", "instrument handle"=w404) -> ("error out"=w397:errorcluster, "instrument handle out"=w398:refnum<k15>)  [unwired: 7 in]
        n215 = call <instrlib>:"niDCPower Configure Voltage Level.vi"("voltage level"="VDD18D, V", "channel name"="0", "instrument handle"=w386) -> ("error out"=w390:errorcluster, "instrument handle out"=w391:refnum<k15>)  [unwired: 7 in]
        n216 = call <instrlib>:"niDCPower Configure Output Enabled.vi"("error in (no error)"=w396, "output enabled"="VDD18_ON", "channel name"="0", "instrument handle"=w399) -> ("error out"=w408:errorcluster, "instrument handle out"=w407:refnum<k15>)  [unwired: 6 in]
        n217 = call <instrlib>:"niDCPower Configure Output Enabled.vi"("error in (no error)"=w397, "output enabled"="VDD33_ON", "channel name"="1", "instrument handle"=w398) -> ("error out"=w409:errorcluster, "instrument handle out"=w410:refnum<k15>)  [unwired: 6 in]
        n218 = call <instrlib>:"niDCPower Configure Output Enabled.vi"("error in (no error)"=w390, "output enabled"="VDD18_ON", "channel name"="0", "instrument handle"=w391) -> ("error out"=w382:errorcluster, "instrument handle out"=w383:refnum<k15>)  [unwired: 6 in]
        n219 = call <instrlib>:"niDCPower Measure.vi"("error in (no error)"=w408, "measurement type"=w381, "channel name"="0", "instrument handle"=w407) -> ("measurement"=w374:dbl)  [unwired: 5 in, 2 out]
        "VDD18A_cur, A" <- w374
        n220 = call <instrlib>:"niDCPower Measure.vi"("error in (no error)"=w409, "measurement type"=w381, "channel name"="1", "instrument handle"=w410) -> ("measurement"=w377:dbl)  [unwired: 5 in, 2 out]
        "VDD33A_cur, A" <- w377
        n221 = call <instrlib>:"niDCPower Measure.vi"("error in (no error)"=w382, "measurement type"=w381, "channel name"="0", "instrument handle"=w383) -> ("measurement"=w375:dbl)  [unwired: 5 in, 2 out]
        "VDD18D_cur, A" <- w375
        n222 = Multiply(x=w374, y=1000.0) -> (x*y=→"VDD18A Chart":dbl)
        n223 = Multiply(x=w377, y=1000.0) -> (x*y=→"VDD33A Chart":dbl)
        n224 = Multiply(x=w375, y=1000.0) -> (x*y=→"VDD18D Chart":dbl)
        n225 = local read "ST"() -> (w366:bool)
      }
    }
  }
  n226 = while {
    tunnel: w6 -> [w421]
    tunnel: w9 -> [_]
    shift-right: ["SPI_прошить"] -> _
    shift-left: w7 -> [w420]
    shift-right: [w414] -> _
    shift-left: w7 -> [w416]
    stop <- w422 stop-if-true
    n227 = local read "Стоп"() -> (w422:bool)
    n228 = local read "RESET"() -> (w414:bool)
    n229 = Greater?(x="SPI_прошить", y=w420) -> (0:w418:bool)
    n230 = Greater?(x=w414, y=w416) -> (0:w415:bool)
    n231 = Or(x=w418, y=w415) -> (x .or. y?=w417:bool)
    n232 = case shown="True" w417 {
      tunnel: w421 -> [_ w424]
      frame False {
        n233 = Wait (ms)(milliseconds to wait=u32 1) -> ()  [unwired: 1 out]
      }
      frame True {
        n234 = stacked-sequence {
          tunnel: w424 -> [_ w427 _]
          frame #0 {
            n235 = Wait (ms)(milliseconds to wait=u32 10) -> ()  [unwired: 1 out]
            "REG_WR" <- FALSE ("Прошили регистры")
          }
          frame #1 {
            n236 = for {
              N: 6 ("Numeric") -> [_]
              tunnel: w427 -> [w429]
              i -> [w430]
              n237 = stacked-sequence {
                tunnel: w429 -> [w433 w500 w502 w506]
                tunnel: w430 -> [w431 _ _ _]
                frame #0 {
                  n238 = case shown="1" w431 {
                    tunnel: [w450 w460 w466 w477 w485 w495] -> w443
                    tunnel: "Запись 6 регистров" -> [w448 w456 w464 w473 w482 w491]
                    tunnel: w431 -> [w449 w457 w465 w474 w483 w492]
                    tunnel: [w447 w455 w463 w472 w481 w490] -> w440
                    frame 0, Default {
                      w452 = FALSE ("element")
                      w451 = TRUE
                      # "W 07"
                      # "0"
                      # "7"
                      n239 = Index Array(array=w448, index=w449) -> (element=w447:u32)
                      n240 = Build Array(w451, w451, w451, w452, w452, w452, w452, TRUE) -> (w454:bool[])
                      n241 = Boolean Array To Number(Boolean array=w454) -> (number=w450:u32)
                    }
                    frame 1 {
                      w458 = FALSE ("element")
                      # "W 08"
                      # "0"
                      # "7"
                      n242 = Index Array(array=w456, index=w457) -> (element=w455:u32)
                      n243 = Build Array(w458, w458, w458, TRUE ("element"), w458, w458, w458, TRUE) -> (w462:bool[])
                      n244 = Boolean Array To Number(Boolean array=w462) -> (number=w460:u32)
                    }
                    frame 2 {
                      w469 = FALSE ("element")
                      # "W 09"
                      # "0"
                      # "7"
                      n245 = Index Array(array=w464, index=w465) -> (element=w463:u32)
                      n246 = Build Array(TRUE, w469, w469, TRUE ("element"), w469, w469, w469, TRUE) -> (w471:bool[])
                      n247 = Boolean Array To Number(Boolean array=w471) -> (number=w466:u32)
                    }
                    frame 3 {
                      w475 = FALSE ("element")
                      # "W 0A"
                      # "0"
                      # "7"
                      n248 = Index Array(array=w473, index=w474) -> (element=w472:u32)
                      n249 = Build Array(w475, TRUE, w475, TRUE ("element"), w475, w475, w475, TRUE) -> (w480:bool[])
                      n250 = Boolean Array To Number(Boolean array=w480) -> (number=w477:u32)
                    }
                    frame 4 {
                      w488 = FALSE ("element")
                      w484 = TRUE
                      # "W 0B"
                      # "0"
                      # "7"
                      n251 = Index Array(array=w482, index=w483) -> (element=w481:u32)
                      n252 = Build Array(w484, w484, w488, TRUE ("element"), w488, w488, w488, TRUE) -> (w489:bool[])
                      n253 = Boolean Array To Number(Boolean array=w489) -> (number=w485:u32)
                    }
                    frame 5 {
                      w498 = FALSE ("element")
                      w493 = TRUE
                      # "W 0E"
                      # "0"
                      # "7"
                      n254 = Build Array(FALSE ("element"), w493, w493, TRUE ("element"), w498, w498, w498, TRUE) -> (w499:bool[])
                      n255 = Index Array(array=w491, index=w492) -> (element=w490:u32)
                      n256 = Boolean Array To Number(Boolean array=w499) -> (number=w495:u32)
                    }
                  }
                  n257 = Multiply(x=w443, y=u32 65536) -> (x*y=w441:u32)
                  n258 = xnode "Read/Write Control"("FPGA VI Reference In"=w433, "8(F)/16(T)"=TRUE) -> ("FPGA VI Reference Out"=w432:refnum<k20>)  [unwired: 1 in, 1 out]
                  n259 = Add(x=w441, y=w440) -> (x+y=w439:u32)
                  n260 = Number To Boolean Array(number=w439) -> (Boolean array=w438:bool[])
                  n261 = Delete From Array(array=w438, length=24, index=0) -> (deleted portion=w435:bool[])  [unwired: 1 out]
                  n262 = xnode "Read/Write Control"("FPGA VI Reference In"=w432, "MOSI"=w435) -> ()  [unwired: 1 in, 2 out]
                  n263 = Wait (ms)(milliseconds to wait=u32 5) -> ()  [unwired: 1 out]
                  n264 = local write "СБОЙ!"(FALSE ("СБОЙ!")) -> ()
                }
                frame #1 {
                  n265 = xnode "Read/Write Control"("FPGA VI Reference In"=w500, "SPI"=TRUE) -> ()  [unwired: 1 in, 2 out]
                }
                frame #2 {
                  n266 = while {
                    tunnel: w502 -> [w505]
                    stop <- w504 stop-if-true
                    n267 = xnode "Read/Write Control"("FPGA VI Reference In"=w505) -> ("SPI_OFF"=w504:bool)  [unwired: 1 in, 2 out]
                    n268 = Wait (ms)(milliseconds to wait=u32 1) -> ()  [unwired: 1 out]
                  }
                }
                frame #3 {
                  n269 = xnode "Read/Write Control"("FPGA VI Reference In"=w506, "SPI"=FALSE) -> ()  [unwired: 1 in, 2 out]
                  n270 = Wait (ms)(milliseconds to wait=u32 5) -> ()  [unwired: 1 out]
                }
              }
            }
          }
          frame #2 {
            n271 = local write "REG_WR"(TRUE ("REG_WR")) -> ()
          }
        }
      }
    }
  }
  n272 = while {
    shift-right: ["SAVE"] -> _
    shift-left: FALSE ("SAVE") -> [w512]
    tunnel: w9 -> [_]
    tunnel: w6 -> [_]
    stop <- w513 stop-if-true
    n273 = local read "Стоп"() -> (w513:bool)
    n274 = Greater?(x="SAVE", y=w512) -> (0:w511:bool)
    n275 = case shown="False" w511 {
      frame False {
        n276 = Wait (ms)(milliseconds to wait=u32 100) -> ()  [unwired: 1 out]
      }
      frame True {
        n277 = local read "Номер образца"() -> (w519:string)
        n278 = Get Date/Time In Seconds() -> (seconds since 1Jan1904=w534:timestamp)
        n279 = Concatenate Strings("Образец_" ("string"), w519) -> (w517:string)
        n280 = Format Date/Time String(time format string (%c)="%H.%M.%S", seconds (now)=w534) -> (date/time string=w538:string)  [unwired: 1 in]
        n281 = Select(t="Светло", s="Светлый (T)\nТемный (F)", f="Темно") -> (s? t:f=w535:string)
        n282 = Build Path(base path="Frames", name or relative path=w517) -> (appended path=w529:path)
        n283 = Concatenate Strings(w538, "_", "ПРИМЕЧАНИЕ", ".tiff" ("element")) -> (w537:string)
        n284 = call <vilib>:"Check if File or Folder Exists.vi"("path"=w529) -> ("file or folder exists?"=w528:bool, "dup path"=w527:path)  [unwired: 8 in, 1 out]
        n285 = case shown="False" w528 {
          tunnel: w527 -> [w544 w545]
          tunnel: [w543 w545] -> w516
          frame False {
            n286 = Create Folder(path (use dialog)=w544) -> (created path=w543:path)  [unwired: 2 in, 2 out]
          }
          frame True {
          }
        }
        n287 = Build Path(base path=w516, name or relative path=w535) -> (appended path=w530:path)
        n288 = call <vilib>:"Check if File or Folder Exists.vi"("path"=w530) -> ("file or folder exists?"=w531:bool, "dup path"=w532:path)  [unwired: 8 in, 1 out]
        n289 = case shown="False" w531 {
          tunnel: w532 -> [w541 w542]
          tunnel: [w540 w542] -> w536
          frame False {
            n290 = Create Folder(path (use dialog)=w541) -> (created path=w540:path)  [unwired: 2 in, 2 out]
          }
          frame True {
          }
        }
        n291 = local read "Image"() -> (w521:T1)
        n292 = Build Path(base path=w536, name or relative path=w537) -> (appended path=w533:path)
        n293 = call-poly "IMAQ Write File 2"("File Path"=w533, "Image"=w521) -> ()  [unwired: 8 in, 2 out]
      }
    }
  }
  n294 = while {
    tunnel: w6 -> [w566]
    tunnel: w9 -> [w568]
    shift-right: [w569] -> _
    shift-left: u8 0 -> [w548]
    tunnel: w6 -> [w565]
    stop <- w567 stop-if-true
    # "Лог сбои"
    # "Проверка на сбои"
    # "Если тиристор, то с 0"
    n295 = local read "RESET"() -> (w546:bool)
    n296 = local read "VDD33_ON"() -> (w547:bool)
    n297 = local read "REG_WR"() -> (w561:bool)
    n298 = local read "Питание"() -> (w560:bool)
    n299 = local read "SEL"() -> (w559:bool)
    n300 = Equal?(x=w548, y=u8 1 ("x")) -> (x = y?=w551:bool)
    n301 = Not(x=w559) -> (.not. x?=w558:bool)
    n302 = Equal?(x=u8 0, y=w548) -> (x = y?=w564:bool)
    n303 = Equal?(x=u8 1, y=w548) -> (x = y?=w563:bool)
    n304 = Equal?(x=u8 3, y=w548) -> (x = y?=w562:bool)
    n305 = Compound Arithmetic op=OR(w564, w563, w562) -> (w554:bool)
    n306 = Select(t=u8 2, s=w551, f=w548) -> (s? t:f=w550:u8)
    n307 = Compound Arithmetic op=AND(w546, w547, w561, w560, w558) -> (w553:bool)
    n308 = case shown="True" w553 {
      tunnel: w550 -> [_ w573]
      tunnel: [u8 0 w582] -> w569
      tunnel: w566 -> [_ w577]
      tunnel: w568 -> [_ w578]
      tunnel: [w571 w580] -> w567
      tunnel: w565 -> [_ _]
      tunnel: w554 -> [_ w574]
      frame False {
        n309 = local read "Стоп"() -> (w571:bool)
        n310 = Wait (ms)(milliseconds to wait=u32 1) -> ()  [unwired: 1 out]
      }
      frame True {
        n311 = Not(x=w574) -> (.not. x?=w575:bool)
        n312 = local read "Стоп"() -> (w580:bool)
        n313 = Increment(x=w573) -> (x+1=w581:u8)
        "GC" <- w581
        n314 = Equal?(x=w581, y=u8 128) -> (x = y?=w576:bool)
        n315 = stacked-sequence {
          seq-local: [_ w601 _ _] -> [_ _ w626 _]
          seq-local: [_ w600 _ _] -> [_ _ w621 _]
          tunnel: w575 -> [w586 w607 _ _]
          tunnel: w578 -> [_ _ _ w648]
          tunnel: w577 -> [w588 w598 _ _]
          tunnel: w576 -> [_ _ _ w647]
          tunnel: w573 -> [w584 w596 w620 _]
          frame #0 {
            n316 = Select(t=u32 65536 ("y"), s=w586, f=u32 256 ("y")) -> (s? t:f=w594:u32)
            n317 = Multiply(x=w584, y=w594) -> (x*y=w595:u32)
            n318 = Number To Boolean Array(number=w595) -> (Boolean array=w593:bool[])
            n319 = xnode "Read/Write Control"("FPGA VI Reference In"=w588, "8(F)/16(T)"=w586) -> ("FPGA VI Reference Out"=w587:refnum<k20>)  [unwired: 1 in, 1 out]
            n320 = xnode "Read/Write Control"("FPGA VI Reference In"=w587, "MOSI"=w593) -> ("FPGA VI Reference Out"=w585:refnum<k20>)  [unwired: 1 in, 1 out]
            n321 = Wait (ms)(milliseconds to wait=u32 1) -> ()  [unwired: 1 out]
            n322 = xnode "Read/Write Control"("FPGA VI Reference In"=w585, "SPI"=TRUE) -> ()  [unwired: 1 in, 2 out]
          }
          frame #1 {
            n323 = xnode "Read/Write Control"("FPGA VI Reference In"=w598, "SPI"=TRUE) -> ("FPGA VI Reference Out"=w597:refnum<k20>)  [unwired: 1 in, 1 out]
            n324 = while {
              tunnel: w597 -> [w617]
              tunnel: [w615] -> w611
              stop <- w616 stop-if-true
              n325 = xnode "Read/Write Control"("FPGA VI Reference In"=w617) -> ("FPGA VI Reference Out"=w615:refnum<k20>, "SPI_OFF"=w616:bool)  [unwired: 1 in, 1 out]
              n326 = Wait (ms)(milliseconds to wait=u32 1) -> ()  [unwired: 1 out]
            }
            n327 = Index Array(array="Содержание всех регистров", index=w596) -> (element=w602:u32)
            n328 = xnode "Read/Write Control"("FPGA VI Reference In"=w611) -> ("FPGA VI Reference Out"=w613:refnum<k20>, "MISO"=w609:bool[])  [unwired: 1 in, 1 out]
            "SPI_OUT" <- w609
            n329 = Select(t=16, s=w607, f=8) -> (s? t:f=w604:i32)
            n330 = xnode "Read/Write Control"("FPGA VI Reference In"=w613, "SPI"=FALSE) -> ()  [unwired: 1 in, 2 out]
            n331 = Delete From Array(array=w609, length=w604, index=0) -> (deleted portion=w603:bool[])  [unwired: 1 out]
            n332 = Boolean Array To Number(Boolean array=w603) -> (number=w600:u16)
            n333 = Not Equal?(x=w600, y=w602) -> (x != y?=w601:bool)
            "COUNT" <- w596
          }
          frame #2 {
            n334 = local read "SEL"() -> (w631:bool)
            n335 = local read "RESET"() -> (w619:bool)
            n336 = local read "REG_WR"() -> (w618:bool)
            n337 = Search 1D Array(1D array="МАСКИРУЕМ", element=w620, start index (0)=0) -> (index of element=w630:i32)
            n338 = Not(x=w631) -> (.not. x?=w624:bool)
            n339 = Greater?(x=w630, y=-1) -> (0:w623:bool)
            n340 = Compound Arithmetic op=AND(w626, "ПРОВЕРКА СБОЕВ?", w624, w623, w619, w618) -> (w622:bool)
            n341 = case shown="True" w622 {
              tunnel: w620 -> [_ w637]
              tunnel: w621 -> [_ w636]
              frame False {
                n342 = local write "СБОЙ"("ОК" ("Где сбой")) -> ()
              }
              frame True {
                w633 = " " ("string")
                w642 = i16 0 ("width (-)")
                w643 = i16 0 ("width (-)")
                n343 = local read "Сбои"() -> (w645:i32)
                n344 = Number To Fractional String(number=w637, width (-)=w643, precision (6)=w643) -> (F-format string=w640:string)  [unwired: 1 in]
                n345 = Number To Fractional String(number=w636, width (-)=w642, precision (6)=w642) -> (F-format string=w634:string)  [unwired: 1 in]
                n346 = Increment(x=w645) -> (x+1=→"Сбои":i32)
                n347 = Concatenate Strings("#" ("string"), w640, w633, "=" ("string"), w633, w634) -> (→"СБОЙ" →"ПОСЛЕДНИЙ СБОЙ":string)
                "СБОЙ!" <- TRUE ("СБОЙ!")
              }
            }
          }
          frame #3 {
            w653 = i16 0 ("width (-)")
            w652 = "\t"
            # "Пишет, в каком регистре произошел сбой"
            n348 = local read "СБОЙ!"() -> (w646:bool)
            n349 = local read "Сбои"() -> (w656:i32)
            n350 = And(x=w646, y=w647) -> (x .and. y?=w649:bool)
            n351 = case shown="True" w649 {
              frame False {
              }
              frame True {
                n352 = flat-sequence {
                  frame #0 {
                    n353 = local write "RESET"(FALSE ("RESET")) -> ()
                  }
                  frame #1 {
                    n354 = Wait (ms)(milliseconds to wait=u32 5) -> ()  [unwired: 1 out]
                  }
                  frame #2 {
                    n355 = local write "RESET"(TRUE ("RESET")) -> ()
                    n356 = Wait (ms)(milliseconds to wait=u32 5) -> ()  [unwired: 1 out]
                  }
                }
              }
            }
            n357 = Number To Fractional String(number=w656, width (-)=w653, precision (6)=w653) -> (F-format string=w655:string)  [unwired: 1 in]
            n358 = Get Date/Time In Seconds() -> (seconds since 1Jan1904=w659:timestamp)
            n359 = local read "СБОЙ"() -> (w654:string)
            n360 = Format Date/Time String(time format string (%c)="%d %H:%M:%S:%3u", seconds (now)=w659) -> (date/time string=w658:string)  [unwired: 1 in]
            n361 = Concatenate Strings(w658, w652, w655, w652, w654, "\r\n") -> (w657:string)
            n362 = Format Into String(initial string=w648, w657) -> ()  [unwired: 2 in, 2 out]
          }
        }
        n363 = Select(t=u8 0, s=w576, f=w581) -> (s? t:f=w582:u8)
      }
    }
  }
  n364 = while {
    tunnel: w5 -> [w671]
    stop <- w667 stop-if-true
    n365 = local read "Стоп"() -> (w667:bool)
    n366 = Wait (ms)(milliseconds to wait=u32 1) -> ()  [unwired: 1 out]
    n367 = xnode "Read/Write Control"("FPGA VI Reference In"=w671, "Автомат"="Автомат", "RESET"="RESET", "Стоп"=w667, "Делитель (24/? = F, Гц)"=u8 2, "Направление бит"=FALSE, "TRIG_2"=u8 100, "TRIG_1"=u8 5) -> ()  [unwired: 1 in, 2 out]
  }
  n368 = xnode "Invoke Method"("FPGA VI Reference In"=w24) -> ()  [unwired: 1 in, 2 out]
  n369 = call <instrlib>:"niDCPower Close.vi"("instrument handle"=w16) -> ()  [unwired: 10 in, 1 out]
  n370 = call <instrlib>:"niDCPower Close.vi"("instrument handle"=w15) -> ()  [unwired: 10 in, 1 out]
  n371 = invoke class="RemoteFCServiceV2" method="Dispose"(reference=w2) -> (reference out=w1:refnum<k24>)  [unwired: 2 in, 2 out]
  n372 = Close Reference(reference=w1) -> ()  [unwired: 1 in, 1 out]
